vi "Process.vi"(0 "write address":u32, 2 "resources":T1={"io resources"={"address"="SRAM\\Address", "read"="SRAM\\Read", "input valid"="SRAM\\Input Valid", "write data"="SRAM\\Write Data", "read data"="SRAM\\Read Data", "read data valid"="SRAM\\Read Data Valid", "ready for input"="SRAM\\Ready for Input"}}, 5 "write data":u64, 7 "write data valid":bool, 9 "read address":u32, 11 "read address valid":bool, 12 "ready for retrieve data (T)":bool=TRUE) -> (4 "retrieve data":u64, 6 "retrieve data valid":bool, 13 "ready for read request":bool, 14 "ready for write":bool)   [LabVIEW 2012, in "niRFRIO SRAM 1.0.0 FPGA.lvlib"]
uses:
  <userlib>/FPGA Library/Code Development/DRAM/RF-RIO/SRAM/1.0.0/FPGA/niRFRIO SRAM 1.0.0 FPGA.lvlib
  <userlib>/FPGA Library/Code Development/DRAM/RF-RIO/SRAM/1.0.0/FPGA/Public/Resources.ctl
  <userlib>/FPGA Library/Code Development/DRAM/RF-RIO/SRAM/1.0.0/FPGA/Public/IO Resources.ctl
  <vilib>/rvi/DataTransferAndStorage/Container/Common/niFpgaContainerMetaDataKey.ctl
  <vilib>/rvi/DataTransferAndStorage/Container/Common/niFpgaContainerState.ctl
  <vilib>/rvi/DataTransferAndStorage/Container/Common/niFpgaDataTypeControl.ctl
  <vilib>/rvi/DataTransferAndStorage/Container/Common/niFpgaContainerImplementationControl.ctl
  <vilib>/rvi/DataTransferAndStorage/Container/Common/niFpgaContainerArbitrationOptionsControl.ctl
  <vilib>/rvi/DataTransferAndStorage/Container/Common/niFpgaTransferTypeControl.ctl
  <vilib>/rvi/DataTransferAndStorage/Container/Common/niFpgaContainerInitializationParameters.ctl
  <vilib>/rvi/Memory/Memory_Types/niFpgaMemoryInterfaceConfiguration.ctl
  <vilib>/rvi/FIFO/Fifo_Types/niFpgaFifoControlLogicControl.ctl
  <vilib>/rvi/DataTransferAndStorage/Container/Common/niFpgaContainerGetUniqueNameForEmu.vi
  <vilib>/rvi/DataTransferAndStorage/Container/Common/niFpgaContainerSetEmuInfo.vi
  <vilib>/rvi/eio/common/nirviEmuReportErrorAndStop.vi
  <vilib>/rvi/LocalResourceManager/LocalResourceManager.xnode
  <instrlib>/RF-RIO/SRAM/1.0.0/FPGA/Private/Write Command.ctl
  <instrlib>/RF-RIO/SRAM/1.0.0/FPGA/Private/Read Command.ctl
  <vilib>/eio/EIONode/EIONode.xnode
  <vilib>/rvi/DataTransferAndStorage/Container/XNode/niFpgaContainer.xnode
  <vilib>/rvi/Memory/Memory_Emulation/niFpgaMemoryEmulationRefIn.vi
  <vilib>/rvi/eio/common/nirviEmuTemplateMethod_errors.vi
  <instrlib>/RF-RIO/FIFO/1.0.0/FPGA/Private/Write U64 FIFO.vi
  <instrlib>/RF-RIO/FIFO/1.0.0/FPGA/Private/Read U64 FIFO.vi
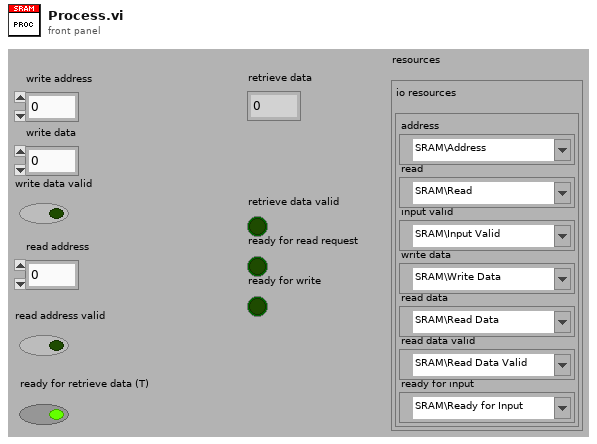
[diagram p1: front panel]
types:
  T1 = typedef "niRFRIO SRAM 1.0.0 FPGA.lvlib/Resources.ctl" = cluster{"io resources":T2}
  T2 = typedef "niRFRIO SRAM 1.0.0 FPGA.lvlib/IO Resources.ctl" = cluster{"address":refnum<k21>, "read":refnum<k21>, "input valid":refnum<k21>, "write data":refnum<k21>, "read data":refnum<k21>, "read data valid":refnum<k21>, "ready for input":refnum<k21>}
  T3 = typedef "niRFRIO SRAM 1.0.0 FPGA.lvlib/Read Command.ctl" = cluster{"address":u32, "valid":bool}
  T4 = typedef "niRFRIO SRAM 1.0.0 FPGA.lvlib/Write Command.ctl" = cluster{"address":u32, "data":u64, "valid":bool}
  T5 = typedef "niRFRIO SRAM 1.0.0 FPGA.lvlib/Command.ctl" = cluster{"address":u32, "write data":u64, "read":bool, "valid":bool}
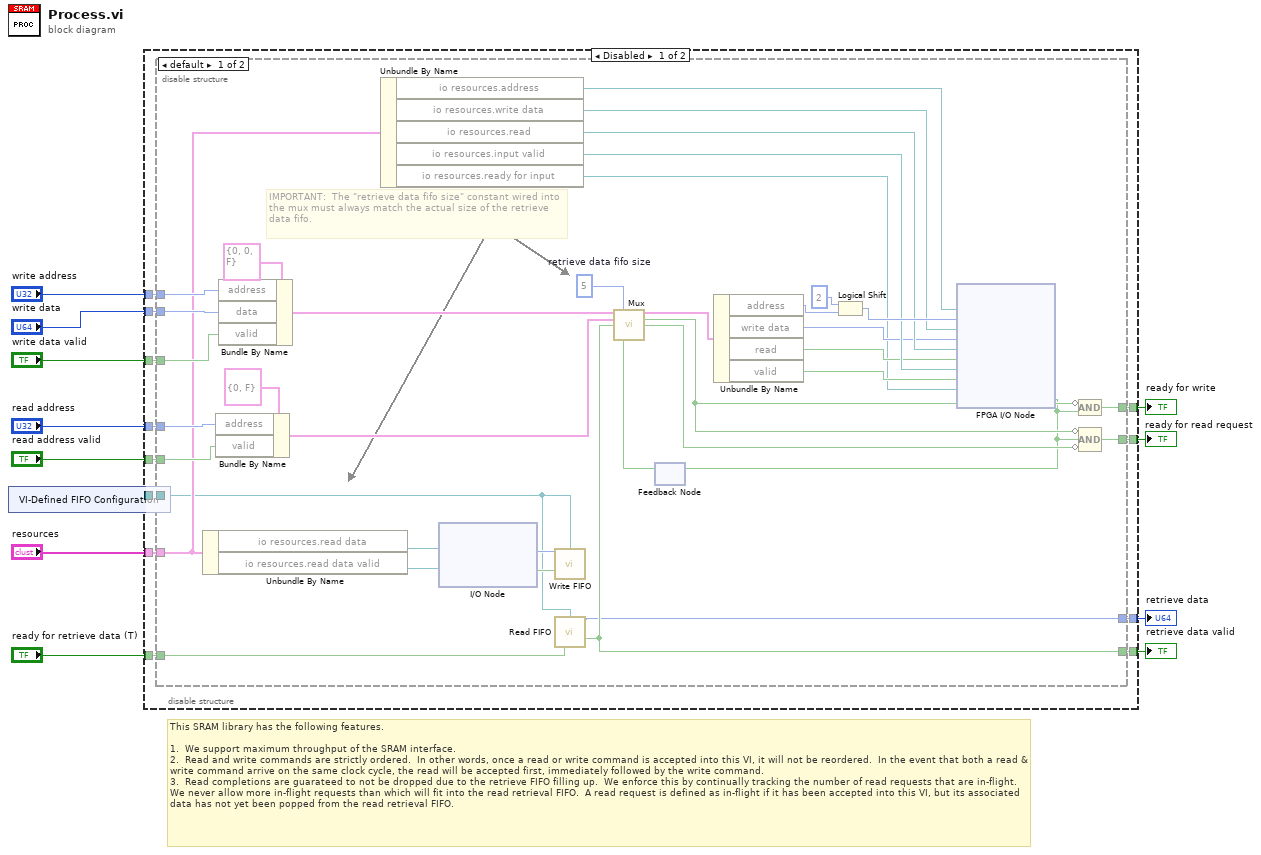
[diagram p0: block diagram]
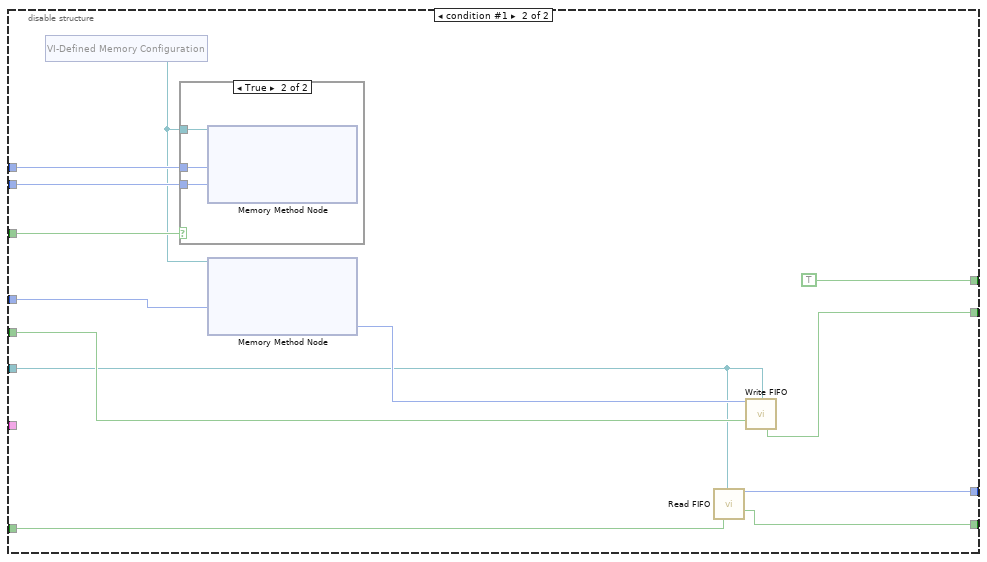
[diagram p2: hidden frame]
diagram:
  # "This SRAM library has the following features.\n\n1.  We support maximum throughput of the SRAM interface.\n2.  Read and write commands are strictly ordered.  In other words, once a read or write command is accepted into this VI, it will not be reordered.  In the event that both a read & write command arrive on the same clock cycle, the read will be accepted first, immediately followed by the write command.\n3.  Read completions are guarateed to not be dropped due to the retrieve FIFO filling up.  We enforce this by continually tracking the number of read requests that are in-flight.  We never allow more in-flight requests than which will fit into the read retrieval FIFO.  A read request is defined as in-flight if it has been accepted into this VI, but its associated data has not yet been popped from the read retrieval FIFO."
  n1 = xnode "VI-Defined FIFO Configuration"() -> ("FIFO Out"=w1:refnum<k21>)
  n2 = disable-structure shown="Disabled" {
    disable-tunnel: "write address" -> [w24 _]
    disable-tunnel: "write data" -> [w23 _]
    disable-tunnel: "write data valid" -> [w22 _]
    disable-tunnel: "read address" -> [w21 _]
    disable-tunnel: "read address valid" -> [w20 _]
    disable-tunnel: [w19 _] -> w7
    disable-tunnel: "ready for retrieve data (T)" -> [w18 _]
    disable-tunnel: [w17 _] -> w5
    disable-tunnel: [w16 _] -> w4
    disable-tunnel: [w15 _] -> w3
    disable-tunnel: "resources" -> [w14 _]
    disable-tunnel: w1 -> [w13 _]
    frame Disabled {
      n3 = disable-structure shown="default" {
        disable-tunnel: w24 -> [w61 w74]
        disable-tunnel: w23 -> [w60 w73]
        disable-tunnel: w22 -> [w59 w72]
        disable-tunnel: w21 -> [w58 w71]
        disable-tunnel: w20 -> [w57 w67]
        disable-tunnel: [w32 w64] -> w19
        disable-tunnel: w18 -> [w36 w62]
        disable-tunnel: [w37 w63] -> w17
        disable-tunnel: [w50 TRUE ("ready for write")] -> w16
        disable-tunnel: [w47 w66] -> w15
        disable-tunnel: w14 -> [w42 _]
        disable-tunnel: w13 -> [w33 w65]
        frame condition #0 (active) {
          w51 = u8 5  # retrieve data fifo size
          # "IMPORTANT:  The \"retrieve data fifo size\" constant wired into the mux must always match the actual size of the retrieve data fifo."
          n4 = Unbundle By Name(w42) -> ("io resources.read data"=w44:refnum<k21>, "io resources.read data valid"=w43:refnum<k21>)
          n5 = Bundle By Name(cluster=T3 {"address"=0, "valid"=FALSE} ("read command"), "address"=w58, "valid"=w57) -> (w53:T3)
          n6 = Bundle By Name(cluster=T4 {"address"=0, "data"=0, "valid"=FALSE} ("write command"), "address"=w61, "data"=w60, "valid"=w59) -> (w55:T4)
          n7 = Unbundle By Name(w42) -> ("io resources.address"=w38:refnum<k21>, "io resources.write data"=w39:refnum<k21>, "io resources.read"=w40:refnum<k21>, "io resources.input valid"=w41:refnum<k21>, "io resources.ready for input"=w26:refnum<k21>)
          n8 = xnode "I/O Node"("FPGA I/O In"=w44, "FPGA I/O In"=w43) -> ("I/O Item"=w35:u64, "I/O Item"=w34:bool)  [unwired: 2 out]
          n9 = call-poly <instrlib>:"Write FIFO.vi"("input data"=w35, "fifo"=w33, "input valid"=w34) -> ()  [unwired: 12 in, 1 out]
          n10 = call-poly <instrlib>:"Read FIFO.vi"("fifo"=w33, "ready for output"=w36) -> ("output data"=w32:u64, "output valid"=w37:bool)  [unwired: 12 in]
          n11 = feedback #1() -> (w52:bool)  [unwired: 1 in]
          n12 = call <instrlib>:"Mux.vi"("write command"=w55, "retrieve data fifo size"=w51, "read command"=w53, "completed read request"=w37, "ready for output"=w52) -> ("command"=w31:T5, "write is pending (1 cycle early)"=w49:bool, "retrieve fifo full (1 cycle early)"=w48:bool)  [unwired: 8 in]
          n13 = Unbundle By Name(w31) -> ("address"=w30:u32, "write data"=w29:u64, "read"=w28:bool, "valid"=w27:bool)
          n14 = Logical Shift(y=i8 2, x=w30) -> (x << y=w45:u32)
          n15 = xnode "FPGA I/O Node"("I/O Item"=w45, "FPGA I/O In"=w38, "I/O Item"=w29, "FPGA I/O In"=w39, "I/O Item"=w28, "FPGA I/O In"=w40, "I/O Item"=w27, "FPGA I/O In"=w41, "FPGA I/O In"=w26) -> ("I/O Item"=w25:bool)  [unwired: 5 out]
          n16 = feedback-in #1(w25) -> ()
          n17 = Compound Arithmetic op=AND(invert w49, w25) -> (w50:bool)
          n18 = Compound Arithmetic op=AND(invert w49, w25, invert w48) -> (w47:bool)
        }
        frame condition #1 {
          n19 = xnode "VI-Defined Memory Configuration"() -> ("Memory Out"=w69:refnum<k21>)
          n20 = case shown="True" w72 {
            tunnel: w69 -> [_ w101]
            tunnel: w74 -> [_ w100]
            tunnel: w73 -> [_ w99]
            frame False {
            }
            frame True {
              n21 = xnode ("Memory Method Node")("Address"=w100, "Data"=w99, "Memory In"=w101) -> ()  [unwired: 1 out]
            }
          }
          n22 = xnode ("Memory Method Node")("Address"=w71, "Memory In"=w69) -> ("Data"=w68:u64)  [unwired: 1 out]
          n23 = call-poly <instrlib>:"Read FIFO.vi"("fifo"=w65, "ready for output"=w62) -> ("output data"=w64:u64, "output valid"=w63:bool)  [unwired: 12 in]
          n24 = call-poly <instrlib>:"Write FIFO.vi"("input data"=w68, "fifo"=w65, "input valid"=w67) -> ("ready for input"=w66:bool)  [unwired: 12 in]
        }
      }
    }
    frame Enabled {
    }
  }
  "ready for read request" <- w3
  "ready for write" <- w4
  "retrieve data valid" <- w5
  "retrieve data" <- w7
